vi "change bundler.vi"(9 "old data type":T1, 10 "new data type":T1, 11 "ElemNms[]":string[](array[string])) -> (3 "elemnames out":string[](array[string]))   [LabVIEW 2013]
uses:
  source/tag/Data Type.ctl
  source/tag/data bus tag description.lvclass
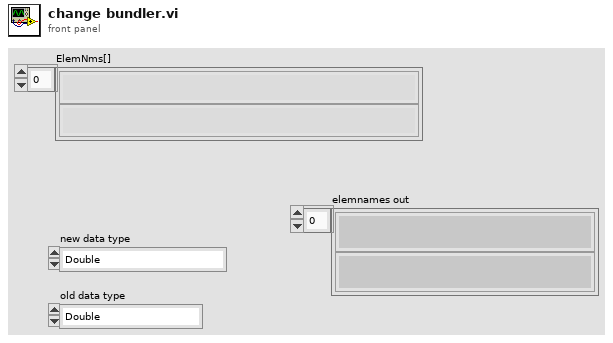
[diagram p1: front panel]
types:
  T1 = typedef "data bus tag description.lvclass/Data Type.ctl" = enum16{"Double", "I64", "Boolean", "Array of Double", "Array of I64", "Variant"}
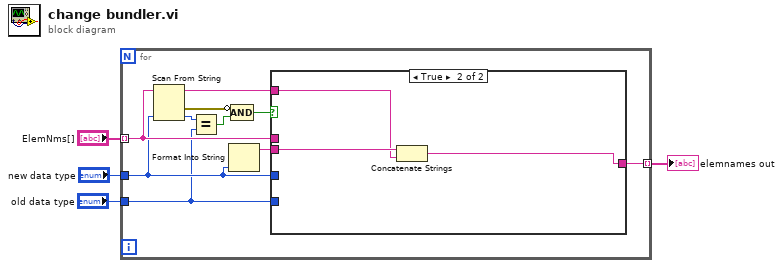
[diagram p0: block diagram]
diagram:
  n1 = for {
    tunnel: "ElemNms[]" -> [w10] mode=indexing
    tunnel: "new data type" -> [w7]
    tunnel: "old data type" -> [w6]
    tunnel: [w9] -> w1 mode=indexing
    n2 = Scan From String(input string=w10, default 1=w7) -> (remaining string=w5:string, error out=w12:errorcluster, output 1=w14:T1)  [unwired: 3 in, 1 out]
    n3 = Equal?(x=w14, y=w6) -> (x = y?=w13:bool)
    n4 = Format Into String(w7) -> (resulting string=w8:string)  [unwired: 3 in, 1 out]
    n5 = Compound Arithmetic op=AND(invert w12, w13) -> (w11:bool)
    n6 = case shown="True" w11 {
      tunnel: w10 -> [w15 _]
      tunnel: [w15 w17] -> w9
      tunnel: w8 -> [_ w18]
      tunnel: w7 -> [_ _]
      tunnel: w6 -> [_ _]
      tunnel: w5 -> [_ w16]
      frame False {
      }
      frame True {
        n7 = Concatenate Strings(w18, w16) -> (w17:string)
      }
    }
  }
  "elemnames out" <- w1
